vi "Write Name.vi"(8 "error in (no error)":errorcluster, 10 "Name":string, 11 "Status Data in":refnum<class "Status Data.lvclass">) -> (0 "error out":errorcluster, 3 "Status Data out":refnum<class "Status Data.lvclass">)   [LabVIEW 2020, in "Status Data.lvclass"]
uses:
  Status Data.lvclass
  Status Data.lvclass/Status Data.ctl
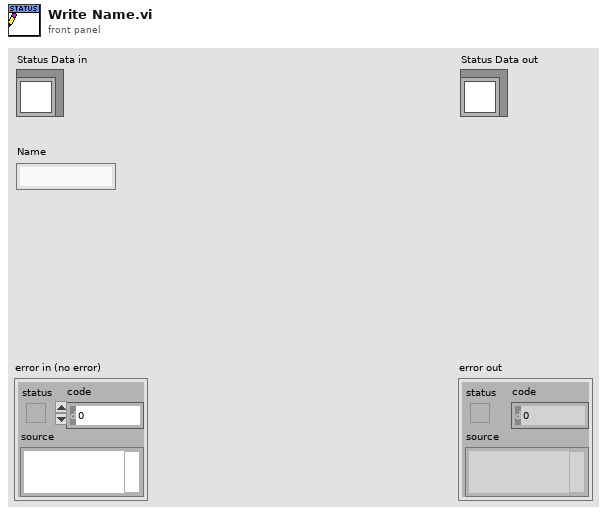
[diagram p1: front panel]
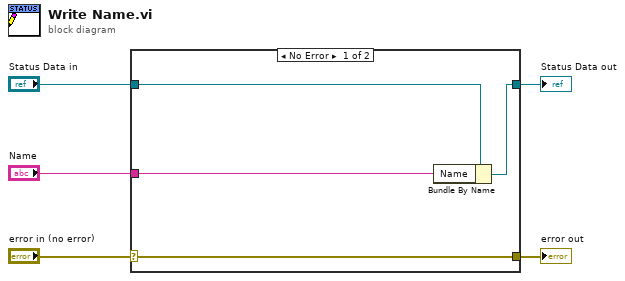
[diagram p0: block diagram]
diagram:
  n1 = case shown="No Error" "error in (no error)" {
    selector: "error in (no error)" -> [w9 w10]
    tunnel: [w9 w10] -> w4
    tunnel: [w7 w11] -> w2
    tunnel: "Status Data in" -> [w8 w11]
    tunnel: "Name" -> [w6 _]
    frame No Error {
      n2 = Bundle By Name(cluster=w8, "Name"=w6) -> (w7:refnum<class "Status Data.lvclass">)
    }
    frame Error {
    }
  }
  "error out" <- w4
  "Status Data out" <- w2
